vi "fileRedGreenRegistrationSave.vi"(1 "filesFolderName":string, 2 "ctrl":dbl[][](array[numeric]), 3 "denormParam":dbl[](array[numeric]), 4 "normParam":dbl[](array[numeric]), 5 "param":dbl[][](array[numeric]), 6 "xy(green)xy(red)":dbl[][](array[numeric])) -> ()   [LabVIEW 2017]
uses:
  <vilib>/Utility/file.llb/Write Delimited Spreadsheet (DBL).vi
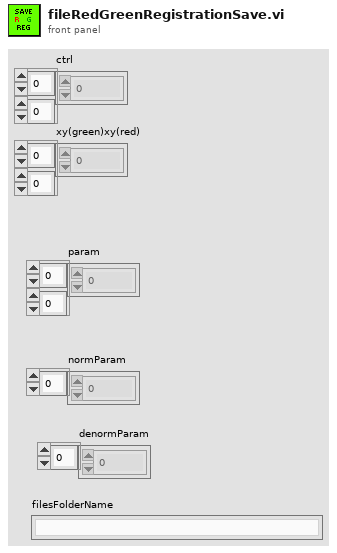
[diagram p1: front panel]
types:
  T1 = enum16{"open", "replace", "create", "open or create", "replace or create", "replace or create with confirmation"}
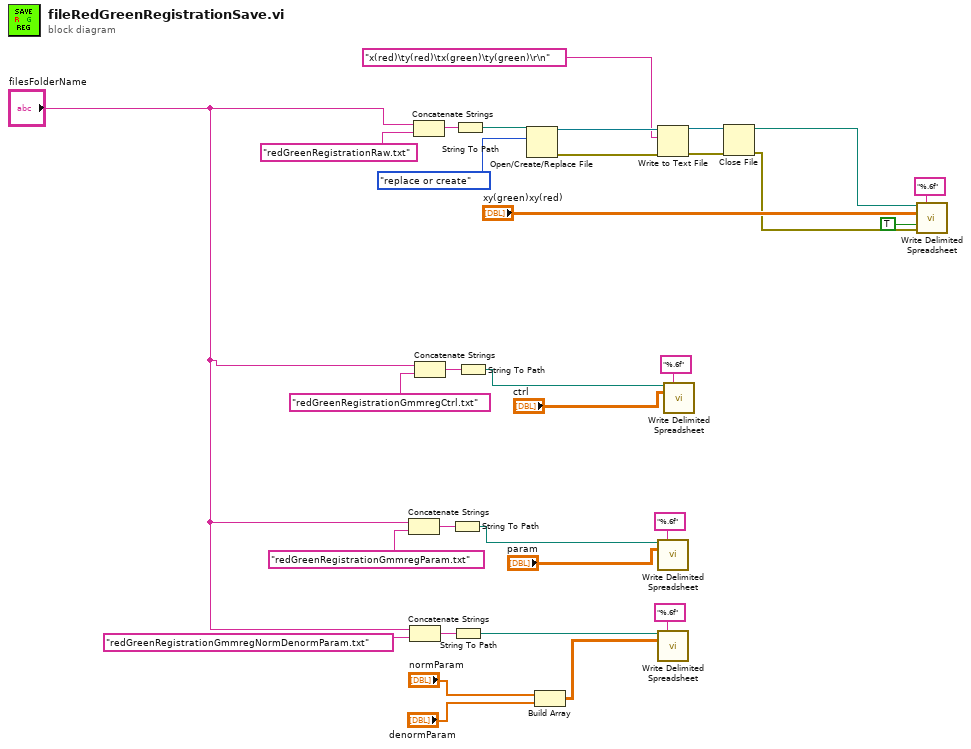
[diagram p0: block diagram]
diagram:
  n1 = Concatenate Strings("filesFolderName", "redGreenRegistrationGmmregParam.txt" ("string")) -> (w16:string)
  n2 = Concatenate Strings("filesFolderName", "redGreenRegistrationGmmregNormDenormParam.txt" ("string")) -> (w9:string)
  n3 = Concatenate Strings("filesFolderName", "redGreenRegistrationRaw.txt" ("string")) -> (w22:string)
  n4 = Concatenate Strings("filesFolderName", "redGreenRegistrationGmmregCtrl.txt" ("string")) -> (w4:string)
  n5 = String To Path(string=w16) -> (path=w15:path)
  n6 = String To Path(string=w9) -> (path=w8:path)
  n7 = String To Path(string=w22) -> (path=w21:path)
  n8 = String To Path(string=w4) -> (path=w5:path)
  n9 = Open/Create/Replace File(file path (use dialog)=w21, operation (0:open)=T1."replace or create") -> (refnum out=w29:refnum<file>, error out=w26:errorcluster)  [unwired: 4 in, 1 out]
  n10 = Build Array("normParam", "denormParam") -> (w7:dbl[][])
  n11 = Write to Text File(file (use dialog)=w29, text="x(red)\ty(red)\tx(green)\ty(green)\r\n", error in=w26) -> (refnum out=w27:refnum<file>, error out=w25:errorcluster)  [unwired: 1 in, 1 out]
  n12 = call-poly <vilib>:"Write Delimited Spreadsheet.vi"("file path (dialog if empty)"=w15, "format (%.3f)"="%.6f", "2D data"="param") -> ()  [unwired: 11 in, 2 out]
  n13 = call-poly <vilib>:"Write Delimited Spreadsheet.vi"("file path (dialog if empty)"=w8, "format (%.3f)"="%.6f", "2D data"=w7) -> ()  [unwired: 11 in, 2 out]
  n14 = call-poly <vilib>:"Write Delimited Spreadsheet.vi"("file path (dialog if empty)"=w5, "format (%.3f)"="%.6f", "2D data"="ctrl") -> ()  [unwired: 11 in, 2 out]
  n15 = Close File(refnum=w27, error in=w25) -> (path=w19:path, error out=w24:errorcluster)
  n16 = call-poly <vilib>:"Write Delimited Spreadsheet.vi"("file path (dialog if empty)"=w19, "format (%.3f)"="%.6f", "2D data"="xy(green)xy(red)", "append to file? (new file:F)"=TRUE, "error in (no error)"=w24) -> ()  [unwired: 9 in, 2 out]
